vi "Move Labels.vi"(8 "error in (no error)":errorcluster, 11 "Objects":refnum<vi>[](array[refnum])) -> (0 "error out":errorcluster, 3 "Objects out":refnum<vi>[](array[refnum]))   [LabVIEW 2019]
doc: "Repositions the visible labels or captions of top-level front panel and block diagram objects to be consistent with the \"Default label position\" settings in Tools > Options. If [Shift] is also pressed, then all objects, including nested objects, are modified. If this shortcut is activated from the front panel, then controls and indicators are modified. If it is activated from the block diagram, then control and indicator terminals are modified. If panel or diagram objects were already selected when this shortcut is activated, only the selected objects that have visible labels or captions are modified.\n\nThe text justification of the modified labels and captions is also modified to be consistent with the new label or caption position.\n\nDefault Shortcut - [T]"
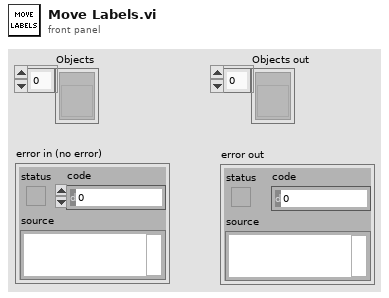
[diagram p1: front panel]
types:
  T1 = typedef "LVRectTypeDef.ctl" = cluster{"Left":i16, "Top":i16, "Right":i16, "Bottom":i16}
  T2 = cluster{"MasterRect":T1, "Label":refnum<vi>, "f":i32, refnum<vi>}
  T3 = enum32{"None", "Size to Fit", "Arrange Horizontally", "Arrange Vertically"}
  T4 = cluster{"Bounds Rect":T1, "Label":refnum<vi>, "f":i32, refnum<vi>}
  T5 = cluster{"Bounds Rect":T1, "Label":refnum<vi>, "right-top":i32, refnum<vi>}
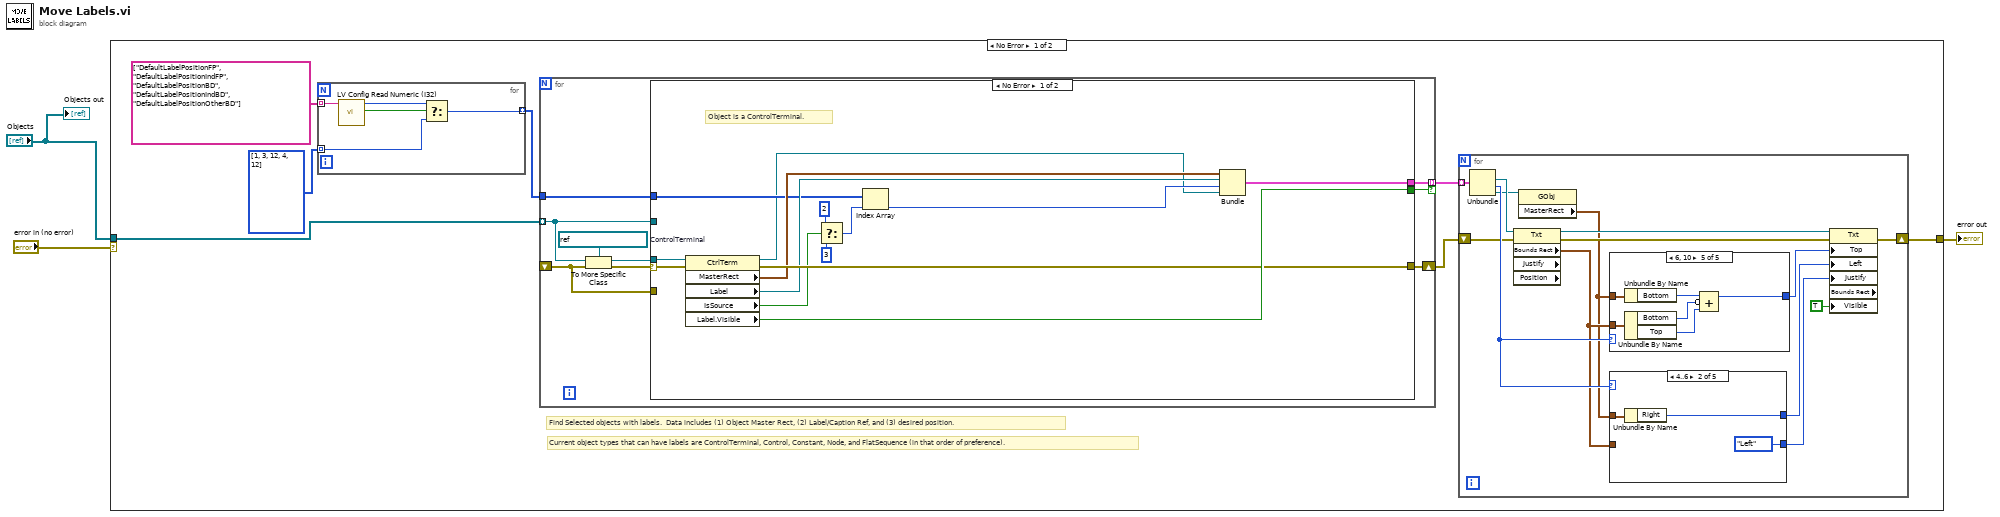
[diagram p0: block diagram]
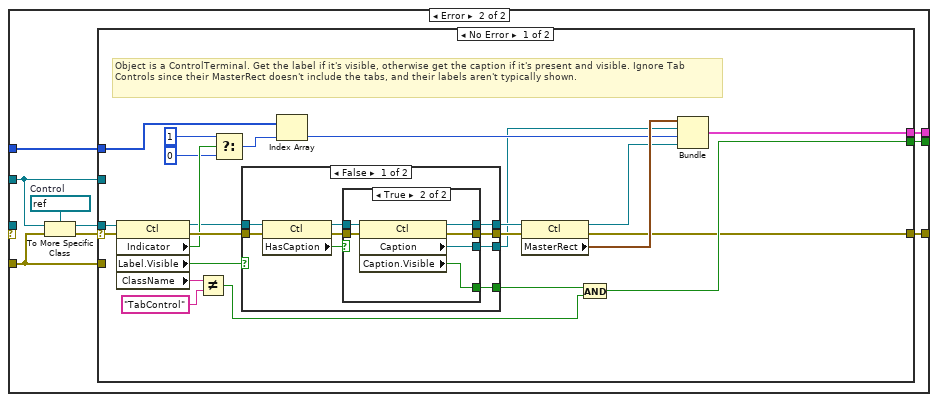
[diagram p2: hidden frame]
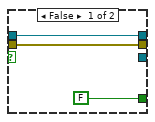
[diagram p3: hidden frame]
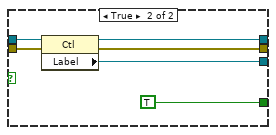
[diagram p4: hidden frame]
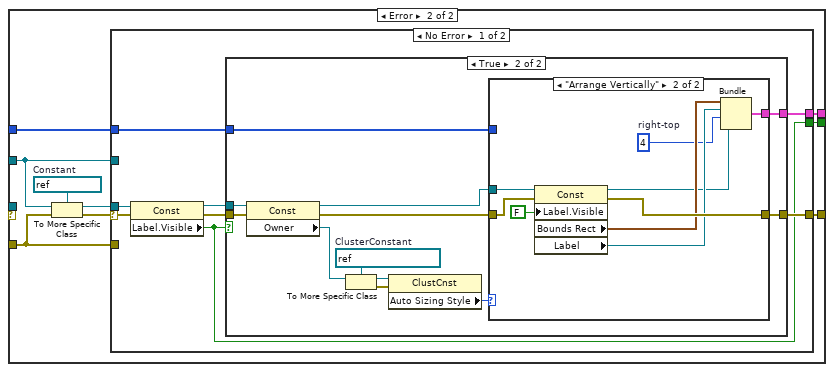
[diagram p5: hidden frame]
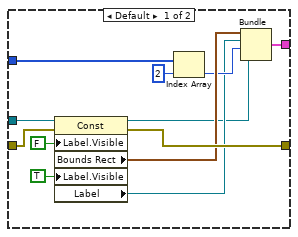
[diagram p7: hidden frame]
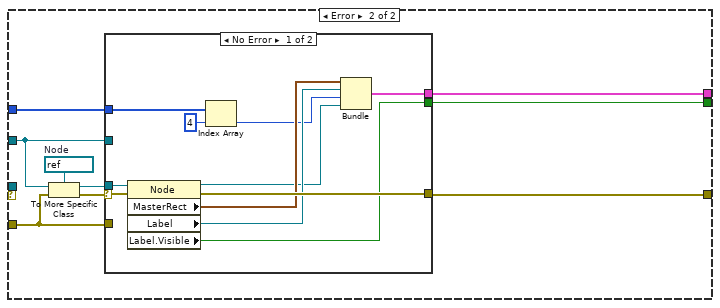
[diagram p8: hidden frame]
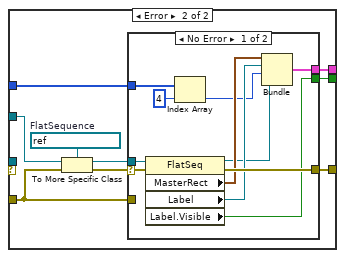
[diagram p9: hidden frame]
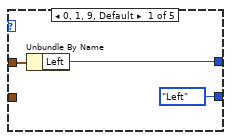
[diagram p11: hidden frame]
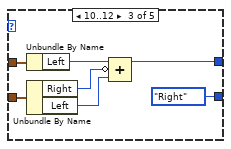
[diagram p12: hidden frame]
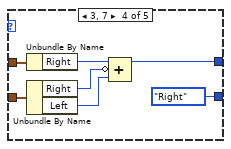
[diagram p13: hidden frame]
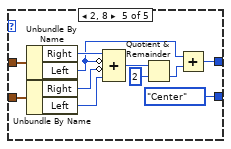
[diagram p14: hidden frame]
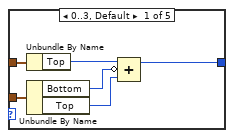
[diagram p15: hidden frame]
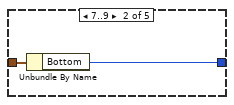
[diagram p16: hidden frame]
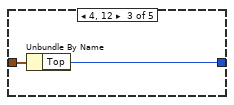
[diagram p17: hidden frame]
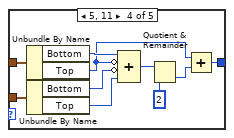
[diagram p18: hidden frame]
diagram:
  n1 = case shown="No Error" "error in (no error)" {
    selector: "error in (no error)" -> [_ w258]
    tunnel: [w5 w258] -> w2
    tunnel: "Objects" -> [w4 _]
    frame No Error {
      # "Current object types that can have labels are ControlTerminal, Control, Constant, Node, and FlatSequence (in that order of preference)."
      # "Find Selected objects with labels.  Data includes (1) Object Master Rect, (2) Label/Caption Ref, and (3) desired position."
      n2 = for {
        tunnel: string[] ["DefaultLabelPositionFP", "DefaultLabelPositionIndFP", "DefaultLabelPositionBD", "DefaultLabelPositionIndBD", "DefaultLabelPositionOtherBD"] -> [w15] mode=indexing
        tunnel: [w12] -> w6 mode=indexing
        tunnel: i32[] [1, 3, 12, 4, 12] -> [w11] mode=indexing
        n3 = call <resource>:"LV Config Read Numeric (I32).vi"("key"=w15) -> ("found?"=w14:bool, "value"=w13:i32)  [unwired: 4 in, 1 out]
        n4 = Select(t=w13, s=w14, f=w11) -> (s? t:f=w12:i32)
      }
      n5 = for {
        shift-right: [w24] -> w7
        shift-left: _ -> [w16]
        tunnel: w4 -> [w22] mode=indexing
        tunnel: [w23] -> w10 mode=indexing if=w18
        tunnel: w6 -> [w17]
        w19 = refnum<vi> refnum  # ControlTerminal
        n6 = To More Specific Class(target class=w19, reference=w22, error in=w16) -> (specific class reference=w20:refnum<vi>, error out=w21:errorcluster)
        n7 = case shown="No Error" w21 {
          selector: w21 -> [w37 _]
          tunnel: [w35 w44] -> w24
          tunnel: w22 -> [_ w43]
          tunnel: [w32 w42] -> w23
          tunnel: w20 -> [w38 _]
          tunnel: [w36 w40] -> w18
          tunnel: w17 -> [w31 w41]
          tunnel: w16 -> [_ w39]
          frame No Error {
            # "Object is a ControlTerminal."
            n8 = property class="CtrlTerm"(reference=w38, error in=w37) -> (reference out=w25:refnum<vi>, error out=w35:errorcluster, "MasterRect"=w34:T1, "Label"=w33:refnum<vi>, "IsSource"=w30:bool, "Label.Visible"=w36:bool)
            n9 = Select(t=2, s=w30, f=3) -> (s? t:f=w27:i32)
            n10 = Index Array(array=w31, index=w27) -> (element=w26:i32)
            n11 = Bundle("MasterRect"=w34, "Label"=w33, "f"=w26, w25) -> (w32:T2)  [unwired: 1 in]
          }
          frame Error {
            w47 = refnum<vi> refnum  # Control
            n12 = To More Specific Class(target class=w47, reference=w43, error in=w39) -> (specific class reference=w46:refnum<vi>, error out=w45:errorcluster)
            n13 = case shown="No Error" w45 {
              selector: w45 -> [w70 _]
              tunnel: w46 -> [w66 _]
              tunnel: [w49 w99] -> w44
              tunnel: w39 -> [_ w100]
              tunnel: w43 -> [_ w98]
              tunnel: [w68 w97] -> w42
              tunnel: w41 -> [w54 w95]
              tunnel: [w51 w96] -> w40
              frame No Error {
                # "Object is a ControlTerminal. Get the label if it's visible, otherwise get the caption if it's present and visible. Ignore Tab Controls since their MasterRect doesn't include the tabs, and their labels aren't typically shown."
                n14 = property class="Ctl"(reference=w66, error in=w70) -> (reference out=w59:refnum<vi>, error out=w67:errorcluster, "Indicator"=w65:bool, "Label.Visible"=w57:bool, "ClassName"=w53:string)
                n15 = Not Equal?(x=w53, y="TabControl") -> (x != y?=w50:bool)
                n16 = Select(t=1, s=w65, f=0) -> (s? t:f=w62:i32)
                n17 = case shown="False" w57 {
                  tunnel: w67 -> [w79 w94]
                  tunnel: [w76 w91] -> w60
                  tunnel: w59 -> [w77 w93]
                  tunnel: [w74 w92] -> w58
                  tunnel: [w72 w90] -> w56
                  tunnel: [w71 TRUE] -> w55
                  frame False {
                    n18 = property class="Ctl"(reference=w77, error in=w79) -> (reference out=w75:refnum<vi>, error out=w78:errorcluster, "HasCaption"=w73:bool)
                    n19 = case shown="True" w73 {
                      tunnel: w78 -> [w81 w88]
                      tunnel: [w81 w87] -> w76
                      tunnel: w75 -> [w82 w86]
                      tunnel: [w82 w85] -> w74
                      tunnel: [_ w84] -> w72
                      tunnel: [FALSE w83] -> w71
                      frame False {
                      }
                      frame True {
                        n20 = property class="Ctl"(reference=w86, error in=w88) -> (reference out=w85:refnum<vi>, error out=w87:errorcluster, "Caption"=w84:refnum<vi>, "Caption.Visible"=w83:bool)
                      }
                    }
                  }
                  frame True {
                    n21 = property class="Ctl"(reference=w93, error in=w94) -> (reference out=w92:refnum<vi>, error out=w91:errorcluster, "Label"=w90:refnum<vi>)
                  }
                }
                n22 = Index Array(array=w54, index=w62) -> (element=w61:i32)
                n23 = property class="Ctl"(reference=w58, error in=w60) -> (reference out=w48:refnum<vi>, error out=w49:errorcluster, "MasterRect"=w69:T1)
                n24 = And(x=w55, y=w50) -> (x .and. y?=w51:bool)
                n25 = Bundle("MasterRect"=w69, "Label"=w56, "f"=w61, w48) -> (w68:T2)  [unwired: 1 in]
              }
              frame Error {
                w103 = refnum<vi> refnum  # Constant
                n26 = To More Specific Class(target class=w103, reference=w98, error in=w100) -> (specific class reference=w101:refnum<vi>, error out=w102:errorcluster)
                n27 = case shown="No Error" w102 {
                  selector: w102 -> [w111 _]
                  tunnel: w100 -> [_ w150]
                  tunnel: w101 -> [w106 _]
                  tunnel: [w110 w151] -> w99
                  tunnel: w98 -> [_ w149]
                  tunnel: [w109 w148] -> w97
                  tunnel: [w104 w147] -> w96
                  tunnel: w95 -> [w108 w146]
                  frame No Error {
                    n28 = property class="Const"(reference=w106, error in=w111) -> (reference out=w105:refnum<vi>, error out=w107:errorcluster, "Label.Visible"=w104:bool)
                    n29 = case shown="True" w104 {
                      tunnel: [w112 w124] -> w110
                      tunnel: [_ w123] -> w109
                      tunnel: w108 -> [_ w122]
                      tunnel: w107 -> [w112 w121]
                      tunnel: w105 -> [_ w119]
                      frame False {
                      }
                      frame True {
                        w116 = refnum<vi> refnum  # ClusterConstant
                        n30 = property class="Const"(reference=w119, error in=w121) -> (reference out=w118:refnum<vi>, error out=w120:errorcluster, "Owner"=w117:refnum<vi>)
                        n31 = To More Specific Class(target class=w116, reference=w117) -> (specific class reference=w114:refnum<vi>, error out=w115:errorcluster)  [unwired: 1 in]
                        n32 = property class="ClustCnst"(reference=w114, error in=w115) -> ("Auto Sizing Style"=w113:T3)  [unwired: 2 out]
                        n33 = case shown="\"Arrange Vertically\"" w113 {
                          tunnel: [w136 w145] -> w124
                          tunnel: [w134 w143] -> w123
                          tunnel: w122 -> [w133 _]
                          tunnel: w120 -> [w127 w140]
                          tunnel: w118 -> [w126 w139]
                          frame Default {
                            n34 = property class="Const"(reference=w126, error in=w127, "Label.Visible"=FALSE, "Label.Visible"=TRUE) -> (reference out=w125:refnum<vi>, error out=w136:errorcluster, "Bounds Rect"=w135:T1, "Label"=w130:refnum<vi>)
                            n35 = Index Array(array=w133, index=2) -> (element=w131:i32)
                            n36 = Bundle("Bounds Rect"=w135, "Label"=w130, "f"=w131, w125) -> (w134:T4)  [unwired: 1 in]
                          }
                          frame "Arrange Vertically" {
                            w138 = 4  # right-top
                            n37 = property class="Const"(reference=w139, error in=w140, "Label.Visible"=FALSE) -> (reference out=w137:refnum<vi>, error out=w145:errorcluster, "Bounds Rect"=w144:T1, "Label"=w142:refnum<vi>)
                            n38 = Bundle("Bounds Rect"=w144, "Label"=w142, "right-top"=w138, w137) -> (w143:T5)  [unwired: 1 in]
                          }
                        }
                      }
                    }
                  }
                  frame Error {
                    w154 = refnum<vi> refnum  # Node
                    n39 = To More Specific Class(target class=w154, reference=w149, error in=w150) -> (specific class reference=w152:refnum<vi>, error out=w153:errorcluster)
                    n40 = case shown="No Error" w153 {
                      selector: w153 -> [w165 _]
                      tunnel: w152 -> [w163 _]
                      tunnel: [w164 w169] -> w151
                      tunnel: w150 -> [_ w170]
                      tunnel: w149 -> [_ w173]
                      tunnel: [w160 w168] -> w148
                      tunnel: [w159 w166] -> w147
                      tunnel: w146 -> [w158 w167]
                      frame No Error {
                        n41 = property class="Node"(reference=w163, error in=w165) -> (reference out=w155:refnum<vi>, error out=w164:errorcluster, "MasterRect"=w162:T1, "Label"=w161:refnum<vi>, "Label.Visible"=w159:bool)
                        n42 = Index Array(array=w158, index=4) -> (element=w156:i32)
                        n43 = Bundle("MasterRect"=w162, "Label"=w161, "f"=w156, w155) -> (w160:T2)  [unwired: 1 in]
                      }
                      frame Error {
                        w174 = refnum<vi> refnum  # FlatSequence
                        n44 = To More Specific Class(target class=w174, reference=w173, error in=w170) -> (specific class reference=w171:refnum<vi>, error out=w172:errorcluster)
                        n45 = case shown="No Error" w172 {
                          selector: w172 -> [w185 _]
                          tunnel: w171 -> [w184 _]
                          tunnel: w170 -> [_ w186]
                          tunnel: [w183 w186] -> w169
                          tunnel: [w180 _] -> w168
                          tunnel: w167 -> [w179 _]
                          tunnel: [w176 _] -> w166
                          frame No Error {
                            n46 = property class="FlatSeq"(reference=w184, error in=w185) -> (reference out=w175:refnum<vi>, error out=w183:errorcluster, "MasterRect"=w182:T1, "Label"=w181:refnum<vi>, "Label.Visible"=w176:bool)
                            n47 = Index Array(array=w179, index=4) -> (element=w177:i32)
                            n48 = Bundle("MasterRect"=w182, "Label"=w181, "f"=w177, w175) -> (w180:T2)  [unwired: 1 in]
                          }
                          frame Error {
                          }
                        }
                      }
                    }
                  }
                }
              }
            }
          }
        }
      }
      n49 = for {
        tunnel: w10 -> [w200] mode=indexing
        shift-right: [w187] -> w5
        shift-left: w7 -> [w197]
        n50 = Unbundle(w200) -> ("Label"=w198:refnum<vi>, "f"=w199:i32, w188:refnum<vi>)  [unwired: 1 out]
        n51 = property class="Txt" props=["Bounds Rect", "Justify", "Position"](reference=w198, error in=w197) -> (reference out=w196:refnum<vi>, error out=w194:errorcluster, "Bounds Rect"=w193:T1)  [unwired: 2 out]
        n52 = property class="GObj"(reference=w188) -> ("MasterRect"=w189:T1)  [unwired: 1 in, 2 out]
        n53 = case shown="6, 10" w199 {
          tunnel: w189 -> [w237 w239 w241 w251 w257]
          tunnel: w193 -> [w236 _ _ w250 w256]
          tunnel: [w232 w238 w240 w246 w252] -> w195
          frame 0..3, Default {
            n54 = Unbundle By Name(w237) -> ("Top"=w235:i16)
            n55 = Unbundle By Name(w236) -> ("Bottom"=w234:i16, "Top"=w233:i16)
            n56 = Compound Arithmetic op=ADD(w235, invert w234, w233) -> (w232:i16)
          }
          frame 7..9 {
            n57 = Unbundle By Name(w239) -> ("Bottom"=w238:i16)
          }
          frame 4, 12 {
            n58 = Unbundle By Name(w241) -> ("Top"=w240:i16)
          }
          frame 5, 11 {
            n59 = Unbundle By Name(w251) -> ("Bottom"=w245:i16, "Top"=w244:i16)
            n60 = Unbundle By Name(w250) -> ("Bottom"=w249:i16, "Top"=w248:i16)
            n61 = Compound Arithmetic op=ADD(w245, invert w244, invert w249, w248) -> (w243:i16)
            n62 = Quotient & Remainder(x=w243, y=i16 2) -> (floor(x/y)=w247:i16)  [unwired: 1 out]
            n63 = Add(x=w244, y=w247) -> (x+y=w246:i16)
          }
          frame 6, 10 {
            n64 = Unbundle By Name(w257) -> ("Bottom"=w255:i16)
            n65 = Unbundle By Name(w256) -> ("Bottom"=w254:i16, "Top"=w253:i16)
            n66 = Compound Arithmetic op=ADD(w255, invert w254, w253) -> (w252:i16)
          }
        }
        n67 = case shown="4..6" w199 {
          tunnel: w189 -> [w203 w206 w213 w220 w229]
          tunnel: w193 -> [_ _ w211 w218 w228]
          tunnel: [w202 w205 w208 w215 w225] -> w192
          tunnel: [enum16{"Left", "Center", "Right"}."Left" ("Justification") enum16{"Left", "Center", "Right"}."Left" ("Justification") enum16{"Left", "Center", "Right"}."Right" ("Justification") enum16{"Left", "Center", "Right"}."Right" ("Justification") enum16{"Left", "Center", "Right"}."Center" ("Justification")] -> w191
          frame 0, 1, 9, Default {
            n68 = Unbundle By Name(w203) -> ("Left"=w202:i16)
          }
          frame 4..6 {
            n69 = Unbundle By Name(w206) -> ("Right"=w205:i16)
          }
          frame 10..12 {
            n70 = Unbundle By Name(w213) -> ("Left"=w212:i16)
            n71 = Unbundle By Name(w211) -> ("Right"=w210:i16, "Left"=w209:i16)
            n72 = Compound Arithmetic op=ADD(w212, invert w210, w209) -> (w208:i16)
          }
          frame 3, 7 {
            n73 = Unbundle By Name(w220) -> ("Right"=w219:i16)
            n74 = Unbundle By Name(w218) -> ("Right"=w217:i16, "Left"=w216:i16)
            n75 = Compound Arithmetic op=ADD(w219, invert w217, w216) -> (w215:i16)
          }
          frame 2, 8 {
            n76 = Unbundle By Name(w229) -> ("Right"=w227:i16, "Left"=w224:i16)
            n77 = Unbundle By Name(w228) -> ("Right"=w230:i16, "Left"=w231:i16)
            n78 = Compound Arithmetic op=ADD(w227, invert w224, invert w230, w231) -> (w222:i16)
            n79 = Quotient & Remainder(x=w222, y=i16 2) -> (floor(x/y)=w226:i16)  [unwired: 1 out]
            n80 = Add(x=w224, y=w226) -> (x+y=w225:i16)
          }
        }
        n81 = property class="Txt" props=["Top", "Left", "Justify", "Bounds Rect", "Visible"](reference=w196, error in=w194, "Top"=w195, "Left"=w192, "Justify"=w191, "Visible"=TRUE) -> (error out=w187:errorcluster)  [unwired: 2 out]
      }
    }
    frame Error {
    }
  }
  "error out" <- w2
  "Objects out" <- "Objects"
